vi "Load Dynamic Insruments.vi"() -> (3 "Instruments":refnum<class "Dynamic Instrument.lvclass">[](array[class]))   [LabVIEW 2016]
uses:
  Dynamic Instrument/Dynamic Instrument/Dynamic Instrument.lvclass
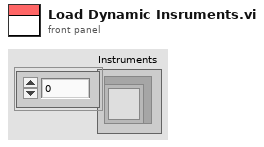
[diagram p1: front panel]
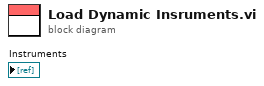
[diagram p0: block diagram]
diagram:
